vi "Get Possible Connections.vi"(8 "error in (no error)":errorcluster, 11 "Hardware Ref in":T2 format="%.0x") -> (0 "error out":errorcluster, 2 "Possible Connections":T1[](array[typedef]), 3 "Hardware Ref out":T2 format="%.0x")   [LabVIEW 2017, in "Routing and Faulting Hardware API.lvlib"]
uses:
  Routing and Faulting Hardware API.lvlib
  <vilib>/NI Veristand/Custom Device API/Custom Device Item Ref.ctl
  Types/Possible Connections for Endpoint.ctl
  NationalInstruments.VeriStand.SystemDefinitionAPI
  Routing and Faulting Hardware API Constants.vi
  <vilib>/NI Veristand/Custom Device API/Custom Device API.lvlib
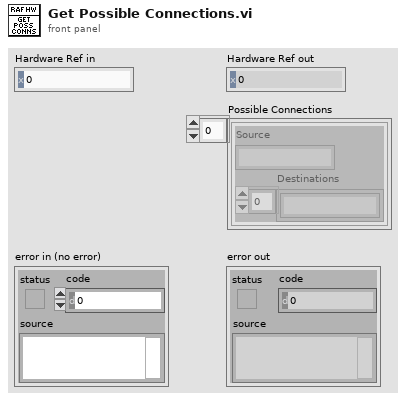
[diagram p1: front panel]
types:
  T1 = typedef "Routing and Faulting Hardware API.lvlib/Possible Connections for Endpoint.ctl" = cluster{"Source":string, "Destinations":string[]}
  T2 = typedef "Custom Device API.lvlib/Custom Device Item Ref.ctl" = u64
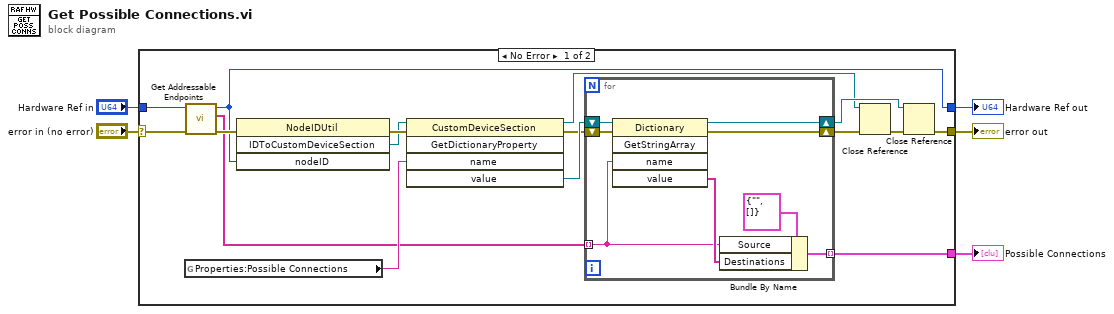
[diagram p0: block diagram]
diagram:
  n1 = case shown="No Error" "error in (no error)" {
    selector: "error in (no error)" -> [w13 w31]
    tunnel: [w20 w31] -> w5
    tunnel: "Hardware Ref in" -> [w11 w30]
    tunnel: [w10 w30] -> w2
    tunnel: [w8 _] -> w1
    frame No Error {
      n2 = global read "Routing and Faulting Hardware API Constants.vi" "Properties:Possible Connections"() -> (w17:string)
      n3 = call "Get Addressable Endpoints.vi"("error in (no error)"=w13, "Hardware Ref in"=w11) -> ("error out"=w12:errorcluster, "Addressable Endpoints"=w9:string[], "Hardware Ref out"=w10:T2)  [unwired: 6 in, 1 out]
      n4 = invoke class="NodeIDUtil" method="IDToCustomDeviceSection"(error in=w12, "nodeID"=w10) -> (error out=w19:errorcluster, "IDToCustomDeviceSection"=w16:refnum<k24>)  [unwired: 2 in, 2 out]
      n5 = invoke class="CustomDeviceSection" method="GetDictionaryProperty"(reference=w16, error in=w19, "name"=w17) -> (reference out=w6:refnum<k24>, error out=w15:errorcluster, "value"=w18:refnum<k24>)  [unwired: 2 in, 2 out]
      n6 = for {
        shift-right: [w22] -> w14
        shift-left: w15 -> [w23]
        shift-right: [w26] -> w7
        shift-left: w18 -> [w27]
        tunnel: w9 -> [w24] mode=indexing
        tunnel: [w28] -> w8 mode=indexing
        n7 = invoke class="Dictionary" method="GetStringArray"(reference=w27, error in=w23, "name"=w24) -> (reference out=w26:refnum<k24>, error out=w22:errorcluster, "value"=w25:string[])  [unwired: 2 in, 2 out]
        n8 = Bundle By Name(cluster=T1 {"Source"="", "Destinations"=[]} ("Possible Connections for Endpoint"), "Source"=w24, "Destinations"=w25) -> (w28:T1)
      }
      n9 = Close Reference(reference=w6, error in (no error)=w14) -> (error out=w21:errorcluster)
      n10 = Close Reference(reference=w7, error in (no error)=w21) -> (error out=w20:errorcluster)
    }
    frame Error {
    }
  }
  "Hardware Ref out" <- w2
  "error out" <- w5
  "Possible Connections" <- w1
